vi "RT_6517B.vi"(1 "Ctl Refnum 2":refnum<vi>, 2 "Ctl Refnum":refnum<vi>, 7 "簇 2":T1, 8 "error in (no error)":errorcluster caption="错误输入（无错误）", 9 "Temp. Adr.":refnum<visa-resource-name> caption="温度计地址", 10 "6517 Adr.":refnum<visa-resource-name> caption="6517地址", 11 "引用句柄输出":refnum<file>) -> (6 "Cluster 2":T2)   [LabVIEW 2017]
panel:
  out "Temperture-Time":cluster{dbl[], dbl[]}(graph)
  out "Present Current (A)":dbl
  out "Time (s)":dbl
  out "Resistivity (ohm·cm)":dbl
  out "电阻 (ohm)":dbl
  in  "电压(V)":dbl
  out "当前温度(°C)":dbl=311.11
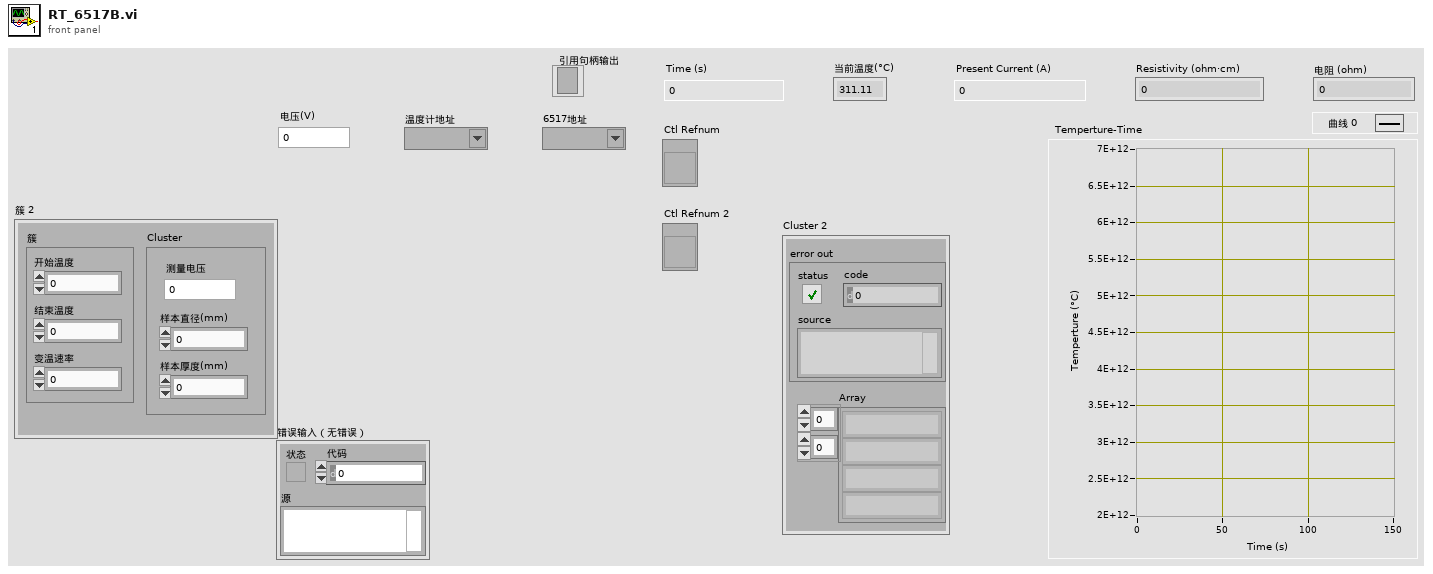
[diagram p1: front panel]
types:
  T1 = cluster{"簇":cluster{"开始温度":dbl, "结束温度":dbl, "变温速率":dbl}, "Cluster":cluster{"测量电压":dbl, "样本直径(mm)":dbl, "样本厚度(mm)":dbl}}
  T2 = cluster{"Array":string[][], "error out":errorcluster}
  T3 = cluster{"测量电压":dbl, "样本直径(mm)":dbl, "样本厚度(mm)":dbl}
  T4 = cluster{dbl, "PV":dbl, "Resistance (ohm)":dbl, dbl}
  T5 = cluster{"Array 2":string[][], "error out":errorcluster}
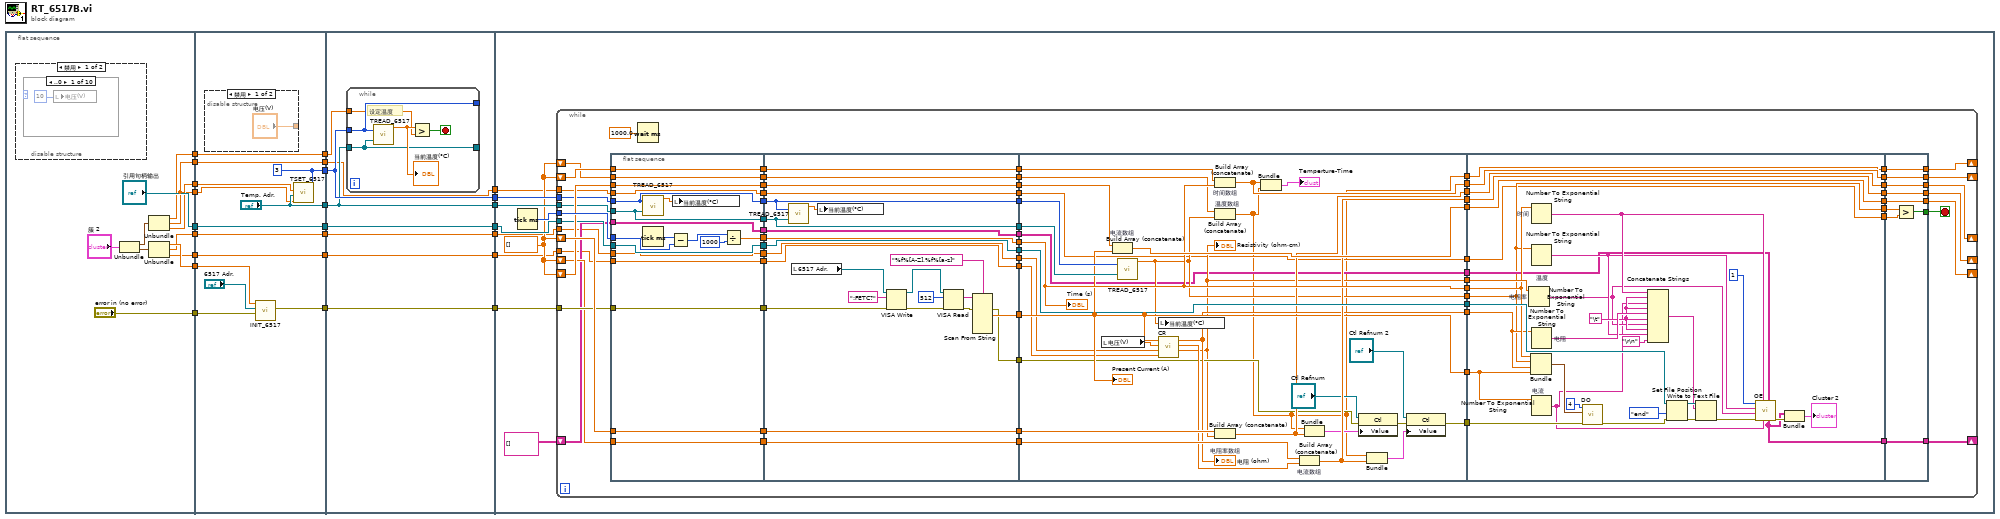
[diagram p0: block diagram]
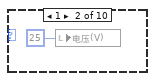
[diagram p2: hidden frame]
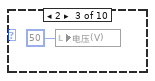
[diagram p3: hidden frame]
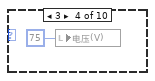
[diagram p4: hidden frame]
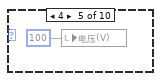
[diagram p5: hidden frame]
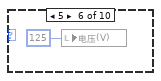
[diagram p6: hidden frame]
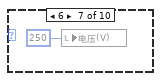
[diagram p7: hidden frame]
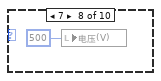
[diagram p8: hidden frame]
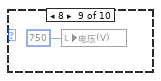
[diagram p9: hidden frame]
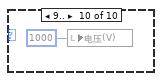
[diagram p10: hidden frame]
diagram:
  n1 = flat-sequence {
    tunnel: ["引用句柄输出"] -> w24
    tunnel: ["error in (no error)"] -> w16
    tunnel: [w30] -> w13
    tunnel: [w29] -> w12
    tunnel: [w27] -> w11
    tunnel: [w28] -> w10
    tunnel: [w27] -> w7
    tunnel: [w26] -> w4
    tunnel: [w25] -> w3
    tunnel: w24 -> [w56]
    tunnel: [w56] -> w23
    tunnel: [w54] -> w22
    tunnel: ["Temp. Adr."] -> w21
    tunnel: [w58] -> w20
    tunnel: w16 -> [w55]
    tunnel: [w52] -> w14
    tunnel: w13 -> [w52]
    tunnel: w12 -> [w51]
    tunnel: w11 -> [w50]
    tunnel: w10 -> [w49]
    tunnel: [w48] -> w8
    tunnel: w7 -> [w48]
    tunnel: [w47] -> w5
    tunnel: w4 -> [w47]
    tunnel: w3 -> [w46]
    tunnel: [w46] -> w2
    tunnel: w23 -> [w67]
    tunnel: w22 -> [w66]
    tunnel: w21 -> [w64]
    tunnel: w20 -> [w65]
    tunnel: [w67] -> w19
    tunnel: [w66] -> w18
    tunnel: [w64] -> w17
    tunnel: [w65] -> w15
    tunnel: w14 -> [w63]
    tunnel: [w62] -> w9
    tunnel: w8 -> [w62]
    tunnel: [w61] -> w6
    tunnel: w5 -> [w61]
    tunnel: w2 -> [w60]
    tunnel: [w60] -> w1
    tunnel: w19 -> [w81]
    tunnel: w18 -> [w80]
    tunnel: w17 -> [w78]
    tunnel: w15 -> [w79]
    tunnel: w9 -> [w75]
    tunnel: w6 -> [w74]
    tunnel: w1 -> [w73]
    frame #0 {
      n2 = disable-structure shown="禁用" {
        frame Disabled {
          n3 = case shown="..0" {
            selector: _ -> [_ _ _ _ _ _ _ _ _ _]
            frame ..0 {
              n4 = local write "电压(V)"(10) -> ()
            }
            frame 1 {
              n5 = local write "电压(V)"(25) -> ()
            }
            frame 2 {
              n6 = local write "电压(V)"(50) -> ()
            }
            frame 3 {
              n7 = local write "电压(V)"(75) -> ()
            }
            frame 4 {
              n8 = local write "电压(V)"(100) -> ()
            }
            frame 5 {
              n9 = local write "电压(V)"(125) -> ()
            }
            frame 6 {
              n10 = local write "电压(V)"(250) -> ()
            }
            frame 7 {
              n11 = local write "电压(V)"(500) -> ()
            }
            frame 8 {
              n12 = local write "电压(V)"(750) -> ()
            }
            frame 9.. {
              n13 = local write "电压(V)"(1000) -> ()
            }
          }
        }
        frame Enabled {
        }
      }
      n14 = Unbundle("簇 2") -> ("簇"=w32:cluster{"开始温度":dbl, "结束温度":dbl, "变温速率":dbl}, "Cluster"=w31:T3)
      n15 = Unbundle(w32) -> ("开始温度"=w30:dbl, "结束温度"=w27:dbl, "变温速率"=w28:dbl)
      n16 = Unbundle(w31) -> ("测量电压"=w29:dbl, "样本直径(mm)"=w26:dbl, "样本厚度(mm)"=w25:dbl)
    }
    frame #1 {
      w58 = i8 3 ("Address No.")
      n17 = disable-structure shown="禁用" {
        disable-tunnel: ["电压(V)" _] -> _
        frame Disabled {
        }
        frame Enabled {
        }
      }
      n18 = call "INIT_6517.vi"("error in (no error)"=w55, "VISA resource name"="6517 Adr.", "Vin"=w51) -> ("error out"=w54:errorcluster)  [unwired: 7 in, 1 out]
      n19 = call "TSET_6517.vi"("Address No."=w58, "T-Ending, C"=w50, "VISA resource name"="Temp. Adr.", "cooling/heating rate, C/min"=w49) -> ()  [unwired: 8 in]
    }
    frame #2 {
      n20 = while {
        tunnel: w64 -> [w69]
        tunnel: w65 -> [w70]
        tunnel: [w70] -> _
        tunnel: [w69] -> _
        tunnel: w63 -> [w68]
        stop <- w71 stop-if-true
        # "设定温度"
        n21 = call "TREAD_6517.vi"("Address No."=w70, "VISA resource name"=w69) -> ("PV"=w72:dbl)  [unwired: 3 out]
        "当前温度(°C)" <- w72
        n22 = Greater?(x=w72, y=w68) -> (0:w71:bool)
      }
    }
    frame #3 {
      w77 = dbl[] []
      n23 = Tick Count (ms)() -> (millisecond timer value=w82:u32)
      n24 = while {
        tunnel: w82 -> [w155]
        shift-right: [w153] -> _
        shift-left: w77 -> [w154]
        shift-right: [w148] -> _
        shift-left: w77 -> [w152]
        shift-right: [w151] -> _
        shift-left: w77 -> [w150]
        tunnel: w81 -> [w147]
        tunnel: w80 -> [w146]
        tunnel: w79 -> [w145]
        tunnel: w78 -> [w144]
        shift-right: [w142] -> _
        shift-left: w77 -> [w143]
        shift-right: [w106] -> _
        shift-left: w77 -> [w103]
        shift-right: [w98] -> _
        shift-left: string[][] [] -> [w93]
        tunnel: w75 -> [w91]
        tunnel: w74 -> [w84]
        tunnel: w73 -> [w83]
        stop <- w149 stop-if-true
        n25 = flat-sequence {
          tunnel: w155 -> [w173]
          tunnel: w146 -> [w160]
          tunnel: w154 -> [w167]
          tunnel: w152 -> [w166]
          tunnel: w150 -> [w165]
          tunnel: w147 -> [w164]
          tunnel: w145 -> [w169]
          tunnel: w144 -> [w168]
          tunnel: w143 -> [w163]
          tunnel: [w160] -> w141
          tunnel: [w167] -> w140
          tunnel: [w166] -> w139
          tunnel: [w165] -> w138
          tunnel: [w164] -> w137
          tunnel: [w170] -> w136
          tunnel: [w163] -> w135
          tunnel: [w169] -> w134
          tunnel: [w168] -> w133
          tunnel: [w162] -> w104
          tunnel: w103 -> [w162]
          tunnel: [w159] -> w94
          tunnel: w93 -> [w159]
          tunnel: [w158] -> w92
          tunnel: w91 -> [w158]
          tunnel: [w157] -> w88
          tunnel: [w156] -> w86
          tunnel: w84 -> [w157]
          tunnel: w83 -> [w156]
          tunnel: w141 -> [w179]
          tunnel: w140 -> [w187]
          tunnel: w139 -> [w186]
          tunnel: w138 -> [w185]
          tunnel: w137 -> [w184]
          tunnel: w136 -> [w183]
          tunnel: w135 -> [w182]
          tunnel: w134 -> [w189]
          tunnel: w133 -> [w188]
          tunnel: [w187] -> w132
          tunnel: [w186] -> w131
          tunnel: [w185] -> w130
          tunnel: [w184] -> w129
          tunnel: [w183] -> w128
          tunnel: [w192] -> w127
          tunnel: [w190] -> w126
          tunnel: [w182] -> w125
          tunnel: [w189] -> w124
          tunnel: [w188] -> w123
          tunnel: [w181] -> w107
          tunnel: w104 -> [w181]
          tunnel: [w178] -> w95
          tunnel: w94 -> [w178]
          tunnel: w92 -> [w177]
          tunnel: [w177] -> w90
          tunnel: w88 -> [w176]
          tunnel: [w176] -> w87
          tunnel: w86 -> [w175]
          tunnel: [w175] -> w85
          tunnel: w132 -> [w231]
          tunnel: w131 -> [w230]
          tunnel: w130 -> [w229]
          tunnel: w129 -> [w222]
          tunnel: w128 -> [w227]
          tunnel: w127 -> [w218]
          tunnel: w126 -> [w208]
          tunnel: w125 -> [w226]
          tunnel: w124 -> [w224]
          tunnel: w123 -> [w223]
          tunnel: [w220] -> w122
          tunnel: [w214] -> w121
          tunnel: [w228] -> w120
          tunnel: [w222] -> w119
          tunnel: [w227] -> w118
          tunnel: [w205] -> w117
          tunnel: [w218] -> w116
          tunnel: [w209] -> w115
          tunnel: [w202] -> w114
          tunnel: [w219] -> w108
          tunnel: w107 -> [w221]
          tunnel: [w215] -> w102
          tunnel: [w213] -> w101
          tunnel: [w204] -> w96
          tunnel: w95 -> [w204]
          tunnel: w90 -> [w203]
          tunnel: [w203] -> w89
          tunnel: w87 -> [w201]
          tunnel: w85 -> [w200]
          tunnel: w122 -> [w258]
          tunnel: w121 -> [w257]
          tunnel: w120 -> [w256]
          tunnel: w119 -> [w264]
          tunnel: w118 -> [w250]
          tunnel: w117 -> [w259]
          tunnel: w116 -> [w248]
          tunnel: w115 -> [w245]
          tunnel: w114 -> [w255]
          tunnel: [w258] -> w113
          tunnel: [w257] -> w112
          tunnel: [w256] -> w111
          tunnel: [w233] -> w110
          tunnel: [w255] -> w109
          tunnel: w108 -> [w254]
          tunnel: [w254] -> w105
          tunnel: w102 -> [w249]
          tunnel: w101 -> [w233]
          tunnel: [w232] -> w100
          tunnel: [w235] -> w97
          tunnel: w96 -> [w237]
          tunnel: w89 -> [w232]
          tunnel: [w271] -> w153
          tunnel: [w270] -> w148
          tunnel: [w269] -> w151
          tunnel: [w272] -> w149
          tunnel: [w268] -> w142
          tunnel: w113 -> [w271]
          tunnel: w112 -> [w270]
          tunnel: w111 -> [w269]
          tunnel: w110 -> [w273]
          tunnel: w109 -> [w268]
          tunnel: [w267] -> w106
          tunnel: w105 -> [w267]
          tunnel: w100 -> [w266]
          tunnel: [w265] -> w98
          tunnel: w97 -> [w265]
          frame #0 {
            n26 = call "TREAD_6517.vi"("Address No."=w169, "VISA resource name"=w168) -> ("PV"=w161:dbl)  [unwired: 3 out]
            n27 = Tick Count (ms)() -> (millisecond timer value=w174:u32)
            n28 = Subtract(x=w174, y=w173) -> (x-y=w172:u32)
            n29 = local write "当前温度(°C)"(w161) -> ()
            n30 = Divide(x=w172, y=u32 1000) -> (x/y=w170:dbl)
          }
          frame #1 {
            n31 = call "TREAD_6517.vi"("Address No."=w189, "VISA resource name"=w188) -> ("PV"=w180:dbl)  [unwired: 3 out]
            n32 = local read "6517 Adr."() -> (w199:refnum<visa-resource-name>)
            n33 = local write "当前温度(°C)"(w180) -> ()
            n34 = VISA Write(VISA resource name=w199, write buffer=":FETC?" ("写入缓冲区"), error in (no error)=w179) -> (VISA resource name out=w196:refnum<visa-resource-name>, error out=w197:errorcluster)  [unwired: 1 out]
            n35 = VISA Read(VISA resource name=w196, byte count=u32 512 ("字节总数"), error in (no error)=w197) -> (read buffer=w194:string, error out=w191:errorcluster)  [unwired: 2 out]
            n36 = Scan From String(format string="%f%[A-Z],%f%[a-z]" ("格式字符串"), input string=w194, error in=w191) -> (error out=w190:errorcluster, output 1=w192:dbl)  [unwired: 1 in, 9 out]
          }
          frame #2 {
            n37 = local read "电压(V)"() -> (w217:dbl)
            n38 = Build Array (concatenate) "电流数组"(w229, w218) -> (w228:dbl[])
            n39 = call "TREAD_6517.vi"("Address No."=w224, "VISA resource name"=w223) -> ("PV"=w213:dbl)  [unwired: 3 out]
            n40 = local write "当前温度(°C)"(w213) -> ()
            n41 = call "CR.vi"("Sample Thickness (mm)"=w200, "Sample Diameter (mm)"=w201, "电压(V)"=w217, "电流(A)"=w218) -> ("Resistivity (ohm·cm)"=w205:dbl, "Current (A)"=w216:dbl, "Resistance (ohm)"=w215:dbl)  [unwired: 5 in]
            "Resistivity (ohm·cm)" <- w205
            "电阻 (ohm)" <- w215
            n42 = Build Array (concatenate) "时间数组"(w231, w227) -> (w220:dbl[])
            n43 = Build Array (concatenate) "温度数组"(w226, w213) -> (w202:dbl[])
            n44 = Build Array (concatenate) "电阻率数组"(w230, w205) -> (w214:dbl[])
            n45 = Bundle(w220, w202) -> (→"Temperture-Time":cluster{dbl[], dbl[]})  [unwired: 1 out]
            n46 = Build Array (concatenate) "电流数组"(w221, w216) -> (w219:dbl[])
            n47 = Bundle(w202, w214) -> (w206:cluster{dbl[], dbl[]})  [unwired: 1 out]
            n48 = property class="Ctl"(reference="Ctl Refnum", error in=w208, "Value"=w206) -> (error out=w210:errorcluster)  [unwired: 1 out]
            n49 = Bundle(w202, w219) -> (w207:cluster{dbl[], dbl[]})  [unwired: 1 out]
            n50 = property class="Ctl"(reference="Ctl Refnum 2", error in=w210, "Value"=w207) -> (error out=w209:errorcluster)  [unwired: 1 out]
            "Present Current (A)" <- w218
            "Time (s)" <- w227
          }
          frame #3 {
            w251 = "\t"
            n51 = Number To Exponential String "电阻率"(number=w259) -> (E-format string=w240:string)  [unwired: 3 out]
            n52 = Bundle(w250, "PV"=w233, "Resistance (ohm)"=w249, w248) -> (w247:T4)  [unwired: 1 in]
            n53 = Number To Exponential String "时间"(number=w250) -> (E-format string=w242:string)  [unwired: 1 in, 2 out]
            n54 = Number To Exponential String "温度"(number=w233) -> (E-format string=w241:string)  [unwired: 3 out]
            n55 = Number To Exponential String "电阻"(number=w249) -> (E-format string=w253:string)  [unwired: 1 in, 2 out]
            n56 = Number To Exponential String "电流"(number=w248) -> (E-format string=w238:string)  [unwired: 3 out]
            n57 = call "DO.vi"("error in (no error)"=w245, "数据输出"=w247, "功能编号"=4) -> ("error out"=w244:errorcluster)  [unwired: 8 in]
            n58 = Concatenate Strings(w242, w251, w238, w251, w253, w251, w240, w251, w241, "\r\n") -> (w261:string)
            n59 = Set File Position(refnum=w264, from (0:start)=enum16{"start", "end", "current"}."end" ("自（0:起始）"), error in=w244) -> (refnum out=w262:refnum<file>, error out=w260:errorcluster)  [unwired: 1 out]
            n60 = Write to Text File(file (use dialog)=w262, text=w261, error in=w260) -> (error out=w239:errorcluster)  [unwired: 1 in, 2 out]
            n61 = call "OE.vi"("Array"=w237, "String 4"=w238, "String"=w242, "error in (no error)"=w239, "String 3"=w240, "String 2"=w241, "Numeric"=1) -> ("error out"=w236:errorcluster, "Array 2"=w235:string[][])  [unwired: 2 in, 1 out]
            n62 = Bundle("Array 2"=w235, "error out"=w236) -> (→"Cluster 2":T5)  [unwired: 1 in]
          }
          frame #4 {
            n63 = Greater?(x=w273, y=w266) -> (0:w272:bool)
          }
        }
        n64 = Wait (ms)(milliseconds to wait=1000.0 ("y")) -> ()  [unwired: 1 out]
      }
    }
  }
